vi "GermanInfo.vi"(4 "Error In":errorcluster, 7 "Command":string) -> (0 "Error Out":errorcluster, 3 "Response":string)   [LabVIEW 2018]
uses:
  MOKO_LabViewLibrary/MokoLowLevel/MokoLowLovelControl/MLLC_Mode.ctl
  data/GermanInfo.ctl
panel:
  in  "Utility name":string="CSMinfo"
  in  "Error Code":i32=5475
  in  "Settings":cluster{"Saved Data":variant, "Data":T1} {"Data"."Окно с настройками"."scheme" items=["Complete test scheme 1", "Complete test scheme 2", "Complete test scheme 3"]}
  in  "Mode":T2=enum."Check"
  # "CSMinfo"
  # "Default Settings"
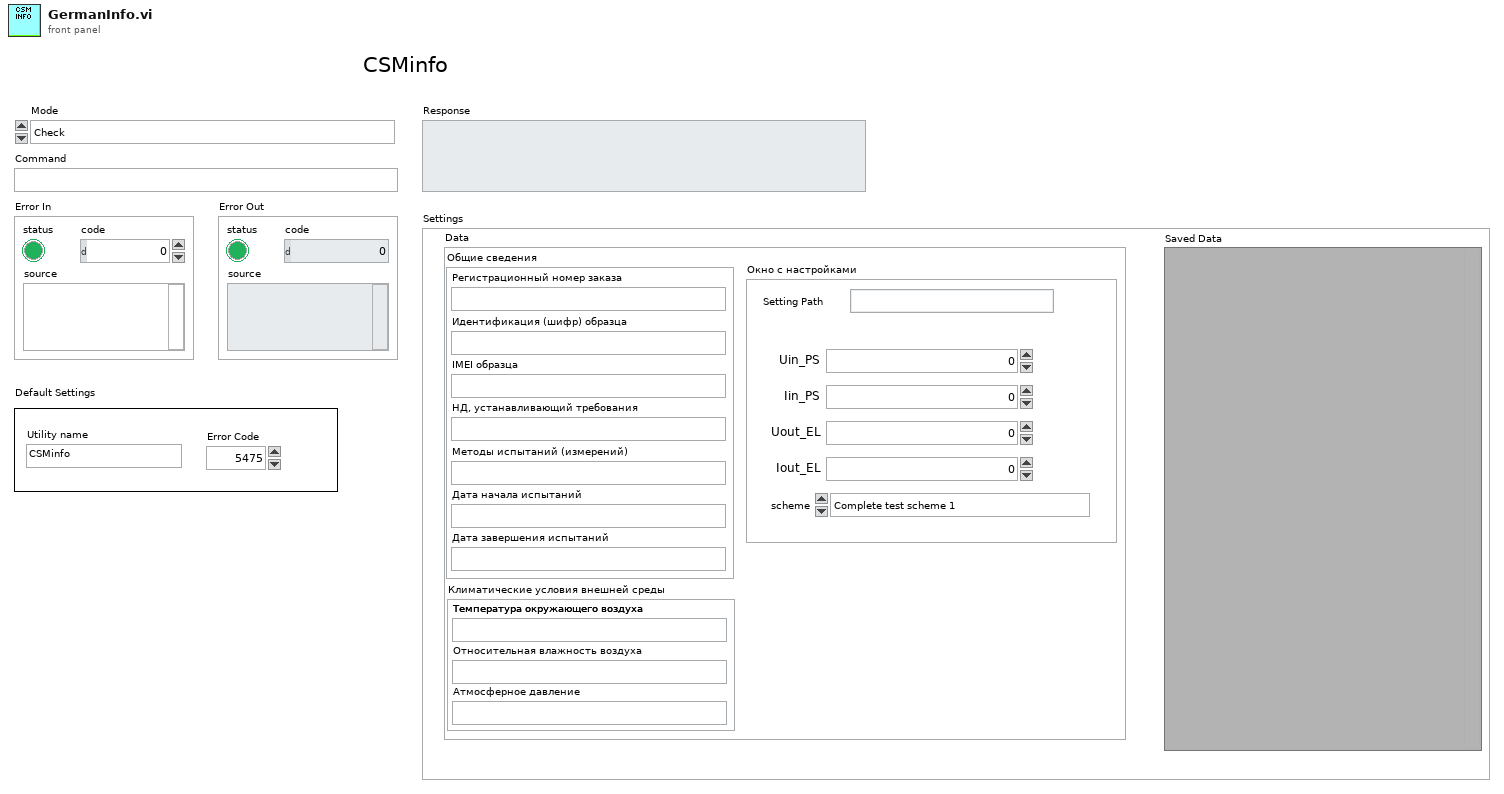
[diagram p1: front panel]
types:
  T1 = typedef "GermanInfo.ctl" = cluster{"Общие сведения":cluster{"Регистрационный номер заказа":string, "Идентификация (шифр) образца":string, "IMEI образца":string, "НД, устанавливающий требования":string, "Методы испытаний (измерений)":string, "Дата начала испытаний":string, "Дата завершения испытаний":string}, "Климатические условия внешней среды":cluster{"Температура окружающего воздуха":string, "Относительная влажность воздуха":string, "Атмосферное давление":string}, "Окно с настройками":cluster{"Uin_PS":dbl, "Setting Path":path, "Iin_PS":dbl, "Uout_EL":dbl, "Iout_EL":dbl, "scheme":u16}}
  T2 = typedef "MLLC_Mode.ctl" = enum16{"get", "set", "close", "Init", "Check"}
  T3 = typedef "MLLC_Error.ctl" = errorcluster
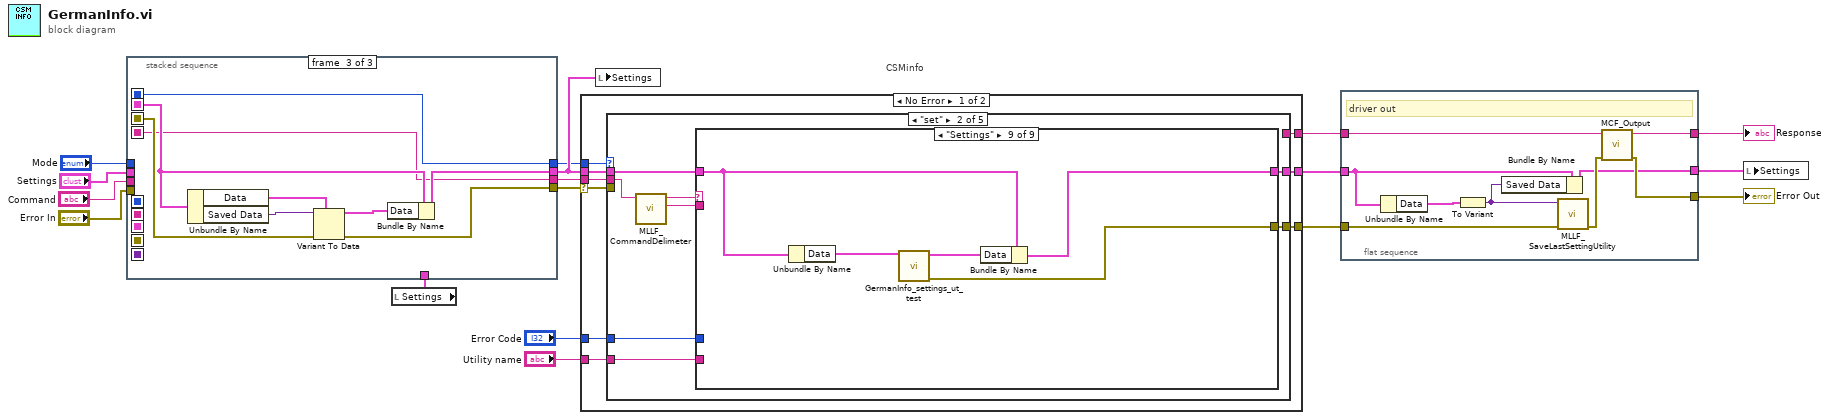
[diagram p0: block diagram]
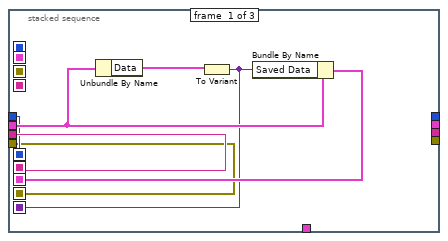
[diagram p2: hidden frame]
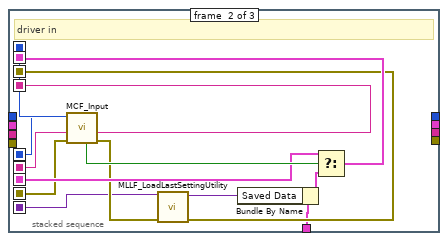
[diagram p3: hidden frame]
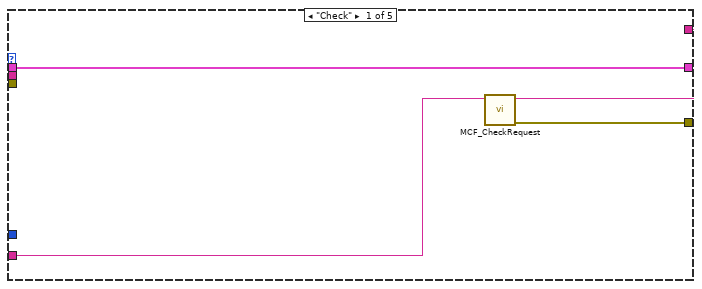
[diagram p4: hidden frame]
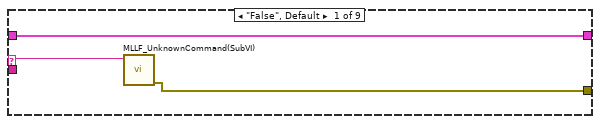
[diagram p5: hidden frame]
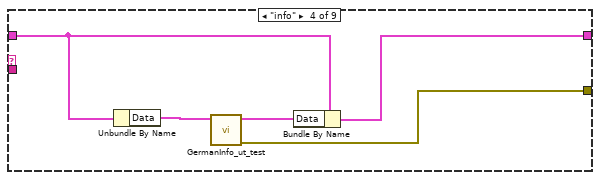
[diagram p8: hidden frame]
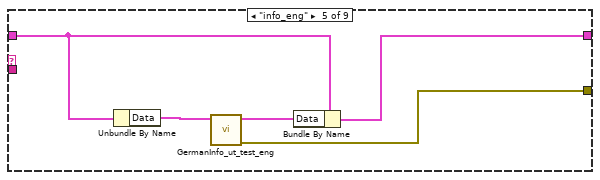
[diagram p9: hidden frame]
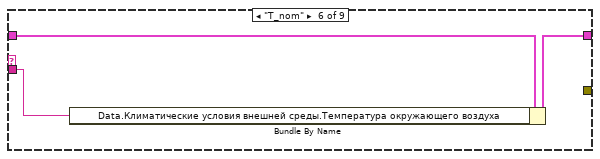
[diagram p10: hidden frame]
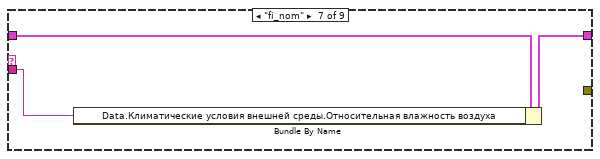
[diagram p11: hidden frame]
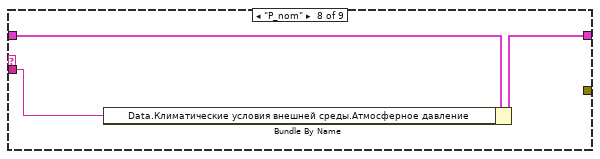
[diagram p12: hidden frame]
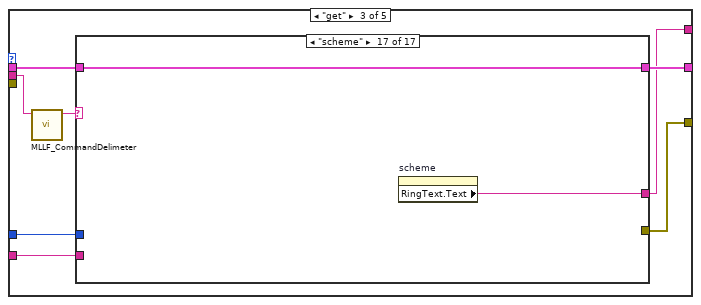
[diagram p13: hidden frame]
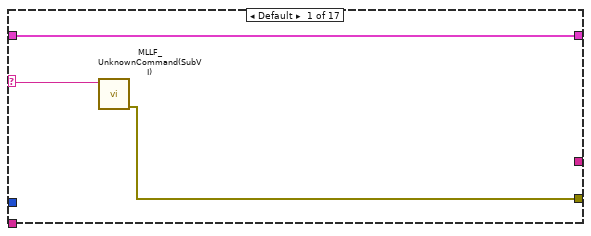
[diagram p14: hidden frame]
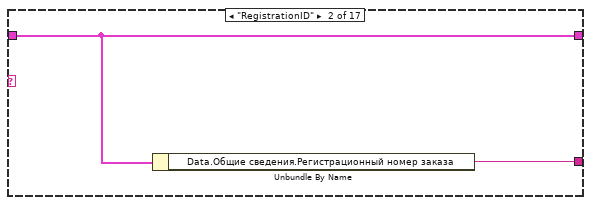
[diagram p15: hidden frame]
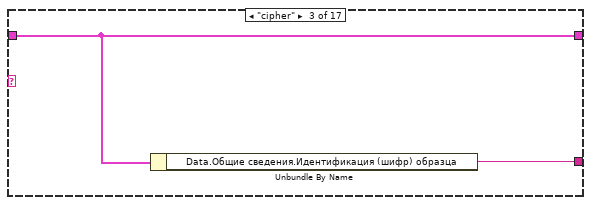
[diagram p16: hidden frame]
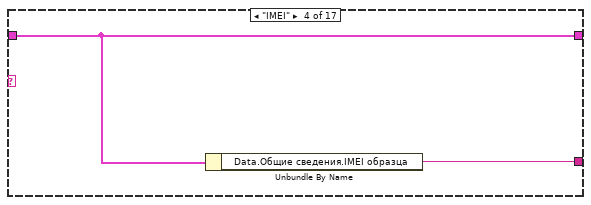
[diagram p17: hidden frame]
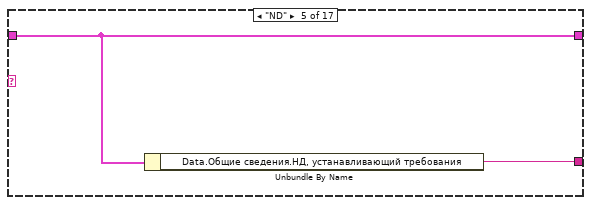
[diagram p18: hidden frame]
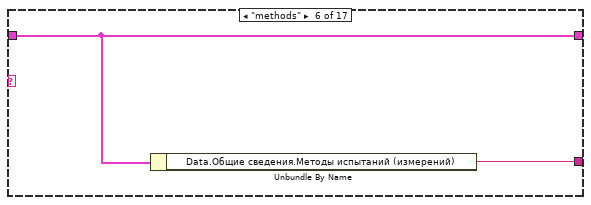
[diagram p19: hidden frame]
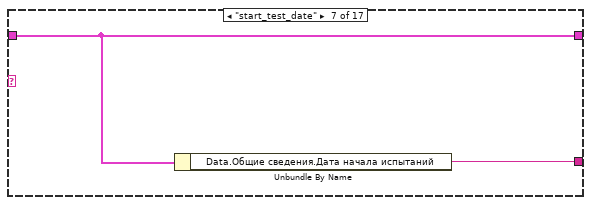
[diagram p20: hidden frame]
diagram:
  # "CSMinfo"
  n1 = local read "Settings"() -> (w12:cluster{"Saved Data":variant, "Data":T1})
  n2 = stacked-sequence {
    seq-local: [w20 _ _] -> [_ w36 _]
    seq-local: [w19 _ _] -> [_ w37 _]
    seq-local: [w22 _ _] -> [_ w32 _]
    seq-local: [w18 _ _] -> [_ w31 _]
    seq-local: [w21 _ _] -> [_ w26 _]
    seq-local: [_ w27 _] -> [_ _ w43]
    seq-local: [_ w38 _] -> [_ _ w40]
    seq-local: [_ w35 _] -> [_ _ w39]
    seq-local: [_ w34 _] -> [_ _ w44]
    tunnel: "Command" -> [w20 _ _]
    tunnel: "Mode" -> [w19 _ _]
    tunnel: "Error In" -> [w18 _ _]
    tunnel: "Settings" -> [w23 _ _]
    tunnel: w12 -> [_ w25 _]
    tunnel: [_ _ w39] -> w8
    tunnel: [_ _ w42] -> w11
    tunnel: [_ _ w41] -> w10
    tunnel: [_ _ w40] -> w9
    frame #0 {
      n3 = Unbundle By Name(w23) -> ("Data"=w24:T1)
      n4 = To Variant(anything=w24) -> (Variant=w21:variant)
      n5 = Bundle By Name(cluster=w23, "Saved Data"=w21) -> (w22:cluster{"Saved Data":variant, "Data":T1})
    }
    frame #1 {
      # "driver in"
      n6 = call "MCF_Input.vi"("Error In"=w31, "Command in"=w36, "Mode in"=w37) -> ("Error Out"=w30:errorcluster, "Command out"=w35:string, "Mode out"=w38:T2, "Boolean"=w33:bool)  [unwired: 5 in]
      n7 = call "MLLF_LoadLastSettingUtility.vi"("Error In"=w30, "Save data in"=w26) -> ("Error Out"=w27:errorcluster, "Save data out"=w29:variant)  [unwired: 8 in]
      n8 = Bundle By Name(cluster=w25, "Saved Data"=w29) -> (w28:cluster{"Saved Data":variant, "Data":T1})
      n9 = Select(t=w32, s=w33, f=w28) -> (s? t:f=w34:cluster{"Saved Data":variant, "Data":T1})
    }
    frame #2 {
      n10 = Unbundle By Name(w44) -> ("Data"=w45:T1, "Saved Data"=w47:variant)
      n11 = Variant To Data(error in=w43, type=w45, Variant=w47) -> (data=w46:T1, error out=w41:errorcluster)
      n12 = Bundle By Name(cluster=w44, "Data"=w46) -> (w42:cluster{"Saved Data":variant, "Data":T1})
    }
  }
  n13 = case shown="No Error" w10 {
    selector: w10 -> [w52 w147]
    tunnel: [w54 w147] -> w16
    tunnel: w9 -> [w56 _]
    tunnel: [w55 _] -> w14
    tunnel: w8 -> [w53 _]
    tunnel: w11 -> [w49 w146]
    tunnel: "Error Code" -> [w51 _]
    tunnel: "Utility name" -> [w50 _]
    tunnel: [w48 w146] -> w15
    frame No Error {
      n14 = case shown="\"set\"" w56 {
        tunnel: [w58 _ w99 _ _] -> w55
        tunnel: [w57 w67 w98 _ _] -> w54
        tunnel: w53 -> [_ w68 w105 _ _]
        tunnel: w52 -> [_ _ _ _ _]
        tunnel: w51 -> [_ w66 w103 _ _]
        tunnel: w50 -> [w59 w63 w102 _ _]
        tunnel: w49 -> [w60 w65 w104 w144 w145]
        tunnel: [w60 w64 w101 w144 w145] -> w48
        frame "Check" {
          n15 = call "MCF_CheckRequest.vi"("Driver Name"=w59) -> ("Error Out"=w57:errorcluster, "Output String"=w58:string)  [unwired: 9 in]
        }
        frame "set" {
          n16 = call "MLLF_CommandDelimeter.vi"("command with param"=w68) -> ("param 1"=w61:string, "command"=w62:string)  [unwired: 6 in, 3 out]
          n17 = case shown="\"Settings\"" w62 {
            selector: w62 -> [w70 _ _ _ _ _ _ _ _]
            tunnel: w61 -> [_ _ _ _ _ w84 w87 w90 _]
            tunnel: [w69 _ _ w78 w83 _ _ _ w97] -> w67
            tunnel: w66 -> [_ _ _ _ _ _ _ _ _]
            tunnel: w65 -> [w71 w72 w73 w77 w82 w86 w89 w92 w95]
            tunnel: [w71 w72 w73 w76 w81 w85 w88 w91 w96] -> w64
            tunnel: w63 -> [_ _ _ _ _ _ _ _ _]
            frame "False", Default {
              n18 = call "MLLF_UnknownCommand(SubVI).vi"("Unknown command"=w70) -> ("error out"=w69:errorcluster)  [unwired: 10 in]
            }
            frame "<----MAIN FUNCTIONS---->" {
            }
            frame "---------ADDITIONAL---------" {
            }
            frame "info" {
              n19 = Unbundle By Name(w77) -> ("Data"=w74:T1)
              n20 = call "GermanInfo_ut_test.vi"("CSMinfo in"=w74) -> ("Error Out"=w78:errorcluster, "CSMinfo out"=w75:T1)  [unwired: 9 in]
              n21 = Bundle By Name(cluster=w77, "Data"=w75) -> (w76:cluster{"Saved Data":variant, "Data":T1})
            }
            frame "info_eng" {
              n22 = Unbundle By Name(w82) -> ("Data"=w79:T1)
              n23 = call "GermanInfo_ut_test_eng.vi"("CSMinfo in"=w79) -> ("Error Out"=w83:errorcluster, "CSMinfo out"=w80:T1)  [unwired: 9 in]
              n24 = Bundle By Name(cluster=w82, "Data"=w80) -> (w81:cluster{"Saved Data":variant, "Data":T1})
            }
            frame "T_nom" {
              n25 = Bundle By Name(cluster=w86, "Data.Климатические условия внешней среды.Температура окружающего воздуха"=w84) -> (w85:cluster{"Saved Data":variant, "Data":T1})
            }
            frame "fi_nom" {
              n26 = Bundle By Name(cluster=w89, "Data.Климатические условия внешней среды.Относительная влажность воздуха"=w87) -> (w88:cluster{"Saved Data":variant, "Data":T1})
            }
            frame "P_nom" {
              n27 = Bundle By Name(cluster=w92, "Data.Климатические условия внешней среды.Атмосферное давление"=w90) -> (w91:cluster{"Saved Data":variant, "Data":T1})
            }
            frame "Settings" {
              n28 = Unbundle By Name(w95) -> ("Data"=w94:T1)
              n29 = call "GermanInfo_settings_ut_test.vi"("Germaninfo in"=w94) -> ("Error Out"=w97:errorcluster, "Germaninfo out"=w93:T1)  [unwired: 9 in]
              n30 = Bundle By Name(cluster=w95, "Data"=w93) -> (w96:cluster{"Saved Data":variant, "Data":T1})
            }
          }
        }
        frame "get" {
          n31 = call "MLLF_CommandDelimeter.vi"("command with param"=w105) -> ("command"=w100:string)  [unwired: 6 in, 4 out]
          n32 = case shown="\"scheme\"" w100 {
            selector: w100 -> [w107 _ _ _ _ _ _ _ _ _ _ _ _ _ _ _ _]
            tunnel: [w106 _ _ _ _ _ _ _ _ _ _ _ _ _ _ _ _] -> w98
            tunnel: w103 -> [_ _ _ _ _ _ _ _ _ _ _ _ _ _ _ _ _]
            tunnel: [w108 w109 w111 w113 w115 w117 w119 w121 w123 w125 w127 w129 w132 w135 w138 w141 w143] -> w101
            tunnel: w104 -> [w108 w109 w111 w113 w115 w117 w119 w121 w123 w125 w127 w129 w132 w135 w138 w141 w143]
            tunnel: w102 -> [_ _ _ _ _ _ _ _ _ _ _ _ _ _ _ _ _]
            tunnel: [_ w110 w112 w114 w116 w118 w120 w122 w124 w126 w128 _ w130 w133 w136 w139 w142] -> w99
            frame Default {
              n33 = call "MLLF_UnknownCommand(SubVI).vi"("Unknown command"=w107) -> ("error out"=w106:errorcluster)  [unwired: 10 in]
            }
            frame "RegistrationID" {
              n34 = Unbundle By Name(w109) -> ("Data.Общие сведения.Регистрационный номер заказа"=w110:string)
            }
            frame "cipher" {
              n35 = Unbundle By Name(w111) -> ("Data.Общие сведения.Идентификация (шифр) образца"=w112:string)
            }
            frame "IMEI" {
              n36 = Unbundle By Name(w113) -> ("Data.Общие сведения.IMEI образца"=w114:string)
            }
            frame "ND" {
              n37 = Unbundle By Name(w115) -> ("Data.Общие сведения.НД, устанавливающий требования"=w116:string)
            }
            frame "methods" {
              n38 = Unbundle By Name(w117) -> ("Data.Общие сведения.Методы испытаний (измерений)"=w118:string)
            }
            frame "start_test_date" {
              n39 = Unbundle By Name(w119) -> ("Data.Общие сведения.Дата начала испытаний"=w120:string)
            }
            frame "completion_test_date" {
              n40 = Unbundle By Name(w121) -> ("Data.Общие сведения.Дата завершения испытаний"=w122:string)
            }
            frame "T_nom" {
              n41 = Unbundle By Name(w123) -> ("Data.Климатические условия внешней среды.Температура окружающего воздуха"=w124:string)
            }
            frame "fi_nom" {
              n42 = Unbundle By Name(w125) -> ("Data.Климатические условия внешней среды.Относительная влажность воздуха"=w126:string)
            }
            frame "P_nom" {
              n43 = Unbundle By Name(w127) -> ("Data.Климатические условия внешней среды.Атмосферное давление"=w128:string)
            }
            frame "------------------- SETTINGS -----------------" {
            }
            frame "Uin", "Uin_PS" {
              n44 = Unbundle By Name(w132) -> ("Data.Окно с настройками.Uin_PS"=w131:dbl)
              n45 = Format Value(value (0)=w131) -> (output string=w130:string)  [unwired: 2 in]
            }
            frame "Iin", "Iin_PS" {
              n46 = Unbundle By Name(w135) -> ("Data.Окно с настройками.Iin_PS"=w134:dbl)
              n47 = Format Value(value (0)=w134) -> (output string=w133:string)  [unwired: 2 in]
            }
            frame "Uout", "Uout_EL" {
              n48 = Unbundle By Name(w138) -> ("Data.Окно с настройками.Uout_EL"=w137:dbl)
              n49 = Format Value(value (0)=w137) -> (output string=w136:string)  [unwired: 2 in]
            }
            frame "Iout", "Iout_EL" {
              n50 = Unbundle By Name(w141) -> ("Data.Окно с настройками.Iout_EL"=w140:dbl)
              n51 = Format Value(value (0)=w140) -> (output string=w139:string)  [unwired: 2 in]
            }
            frame "scheme" {
              n52 = property on="scheme" class="Ring (strict)"() -> ("RingText.Text"=w142:string)  [unwired: 2 in, 2 out]
            }
          }
        }
        frame "close" {
        }
        frame "Init" {
        }
      }
    }
    frame Error {
    }
  }
  n53 = local write "Settings"(w11) -> ()
  n54 = flat-sequence {
    tunnel: [w156] -> w6
    tunnel: [w155] -> w4
    tunnel: w14 -> [w154]
    tunnel: w16 -> [w153]
    tunnel: w15 -> [w149]
    tunnel: [w151] -> w13
    frame #0 {
      # "driver out"
      n55 = Unbundle By Name(w149) -> ("Data"=w148:T1)
      n56 = To Variant(anything=w148) -> (Variant=w150:variant)
      n57 = Bundle By Name(cluster=w149, "Saved Data"=w150) -> (w151:cluster{"Saved Data":variant, "Data":T1})
      n58 = call "MLLF_SaveLastSettingUtility.vi"("error in"=w153, "Saved Data"=w150) -> ("error out"=w152:T3)  [unwired: 8 in, 1 out]
      n59 = call "MCF_Output.vi"("Error In"=w152, "Input"=w154) -> ("Error Out"=w155:errorcluster, "Output"=w156:string)  [unwired: 8 in]
    }
  }
  n60 = local write "Settings"(w13) -> ()
  "Response" <- w6
  "Error Out" <- w4
